vi "Assert ExcuseNotes.vi"() -> ()   [LabVIEW 2015, in "Admin_Actor.lvlib" / "ExcuseNotesHandler.lvclass"]
uses:
  ExcuseNotesHandler.lvclass
  API/_Database/Database.lvclass
  ExcuseNotesHandler.lvclass/ExcuseNotesHandler.ctl
  Admin_Actor.lvlib
panel:
  in  "path":path=path "E:/哈工大竞技机器人队/机器人队管理系统/Database/CRTDatabase.accdb"
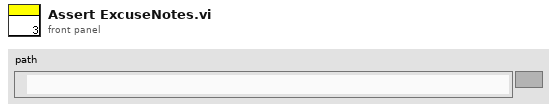
[diagram p1: front panel]
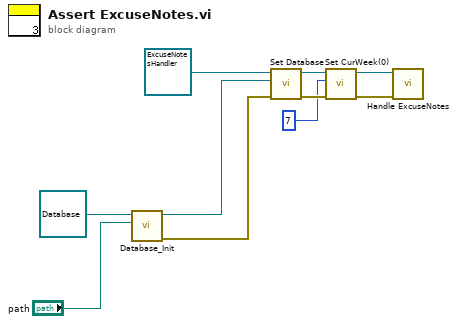
[diagram p0: block diagram]
diagram:
  n1 = call "Database_Init.vi"("path"="path", "object in"=refnum<class "Database.lvclass"> refnum ("Database")) -> ("error out"=w6:errorcluster, "object out"=w7:refnum<class "Database.lvclass">)  [unwired: 8 in]
  n2 = call "Set Database.vi"("error in (no error)"=w6, "Database"=w7, "ExcuseNotes in"=refnum<class "ExcuseNotesHandler.lvclass"> refnum ("Admin_Actor.lvlib:ExcuseNotes.lvclass")) -> ("error out"=w4:errorcluster, "ExcuseNotes out"=w5:refnum<class "ExcuseNotesHandler.lvclass">)  [unwired: 7 in]
  n3 = call "Set CurWeek(0).vi"("error in (no error)"=w4, "CurWeek(0)"=7, "ExcuseNotesHandler in"=w5) -> ("error out"=w2:errorcluster, "ExcuseNotesHandler out"=w3:refnum<class "ExcuseNotesHandler.lvclass">)  [unwired: 7 in]
  n4 = call "Handle ExcuseNotes.vi"("error in (no error)"=w2, "ExcuseNotes.lvclass"=w3) -> ()  [unwired: 8 in, 2 out]
